vi "Get Date Time ISO.vi"(8 "error in (no error)":errorcluster) -> (0 "error out":errorcluster, 1 "ISO 8601 date-time string":string, 2 "current time":timestamp)   [LabVIEW 2019, in "Control Experiment.lvclass"]
uses:
  <userlib>/LevyLab/Transport/Control Experiment/Control Experiment.lvclass
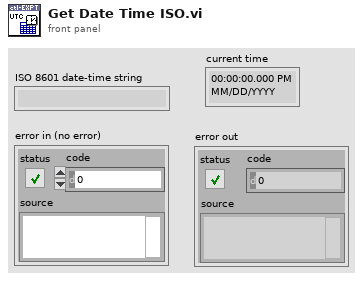
[diagram p1: front panel]
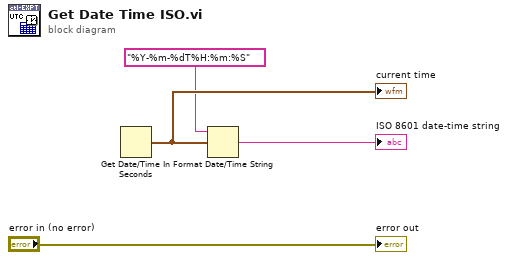
[diagram p0: block diagram]
diagram:
  n1 = Get Date/Time In Seconds() -> (seconds since 1Jan1904=w2:timestamp)
  "current time" <- w2
  n2 = Format Date/Time String(time format string (%c)="%Y-%m-%dT%H:%m:%S", seconds (now)=w2) -> (date/time string=→"ISO 8601 date-time string":string)  [unwired: 1 in]
  "error out" <- "error in (no error)"
